vi "Pause Until Release.vi"(0 "Pause":bool) -> ()   [LabVIEW 2020]
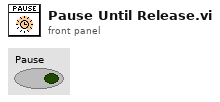
[diagram p1: front panel]
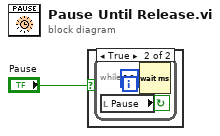
[diagram p0: block diagram]
diagram:
  n1 = case shown="True" "Pause" {
    frame False {
    }
    frame True {
      n2 = while {
        stop <- w3 continue-if-true
        n3 = local read "Pause"() -> (w3:bool)
        n4 = Wait (ms)(milliseconds to wait=u32 10) -> ()  [unwired: 1 out]
      }
    }
  }
